vi "BoydJoya MyFirstFPGA App.vi"() -> ()   [LabVIEW 2011]
uses:
  <vilib>/rvi/eio/common/nirviEmuTemplateMethod_errors.vi
  <vilib>/eio/EIONode/EIONode.xnode
panel:
  in  "Count(mSec)":u32
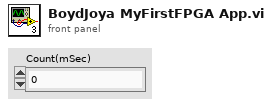
[diagram p1: front panel]
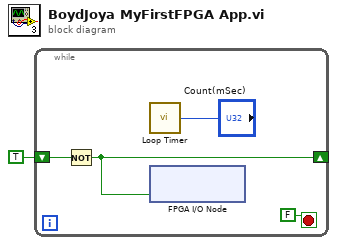
[diagram p0: block diagram]
diagram:
  n1 = while {
    shift-right: [w4] -> _
    shift-left: TRUE -> [w5]
    stop <- FALSE stop-if-true
    n2 = Not(x=w5) -> (.not. x?=w4:bool)
    n3 = call "Loop Timer"("Count(mSec)"="Count(mSec)") -> ()  [unwired: 1 out]
    n4 = xnode "FPGA I/O Node"("FPGA LED"=w4) -> ()  [unwired: 1 in, 1 out]
  }
